vi "Keithley2200series_WaitKeyIccMeas.vi"(0 "VISA Key_In":refnum<visa-resource-name>, 1 "Key":string, 2 "VISA Icc_In":refnum<visa-resource-name>, 3 "error Icc_In":errorcluster) -> (4 "VISA Key_Out":refnum<visa-resource-name>, 6 "Icc, А":string, 7 "Icc, A":dbl, 8 "VISA Icc_Out":refnum<visa-resource-name>, 9 "error Icc_Out":errorcluster)   [LabVIEW 2014]
uses:
  <vilib>/Utility/error.llb/whitespace.ctl
  C:/Users/rad/Desktop/Keithley 2200 Series Power Supplies Ver 1.2 (LV2009)/Keithley 2200 Series/Keithley 2200 Series.lvlib
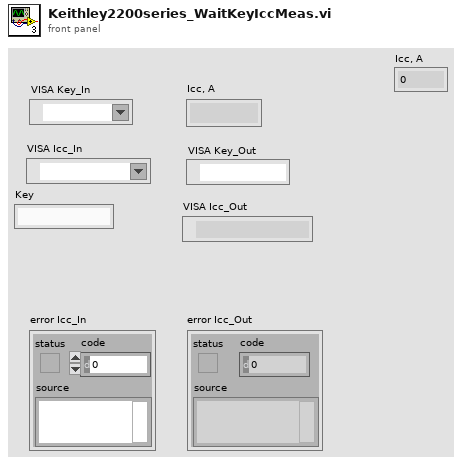
[diagram p1: front panel]
types:
  T1 = typedef "whitespace.ctl" = u16
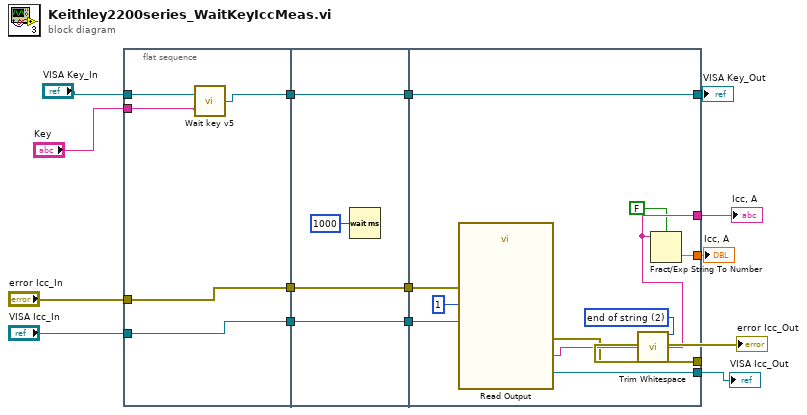
[diagram p0: block diagram]
diagram:
  n1 = flat-sequence {
    tunnel: [w16] -> w6
    tunnel: "VISA Key_In" -> [w18]
    tunnel: [w20] -> w4
    tunnel: "error Icc_In" -> [w20]
    tunnel: [w19] -> w2
    tunnel: "VISA Icc_In" -> [w19]
    tunnel: "Key" -> [w17]
    tunnel: w6 -> [w24]
    tunnel: [w24] -> w5
    tunnel: w4 -> [w23]
    tunnel: [w23] -> w3
    tunnel: w2 -> [w22]
    tunnel: [w22] -> w1
    tunnel: [w32] -> w11
    tunnel: w5 -> [w32]
    tunnel: w3 -> [w31]
    tunnel: w1 -> [w30]
    tunnel: [w29] -> w14
    tunnel: [w28] -> w15
    tunnel: [w27] -> w9
    tunnel: [w26] -> w8
    frame #0 {
      n2 = call "Wait key v5.vi"("Key"=w17, "VISA Refnum in"=w18) -> ("VISA Refnum out"=w16:refnum<visa-resource-name>)
    }
    frame #1 {
      n3 = Wait (ms)(milliseconds to wait=u32 1000) -> ()  [unwired: 1 out]
    }
    frame #2 {
      w34 = T1 2 items=["both", "start of string", "end of string"] ("location (both)")
      n4 = call "Read Output.vi"("VISA resource name"=w30, "Measurement Function (0:Voltage)"=1, "error in (no error)"=w31) -> ("VISA resource name out"=w29:refnum<visa-resource-name>, "Measurement"=w33:string, "error out"=w28:errorcluster)  [unwired: 10 in]
      n5 = call <vilib>:"Trim Whitespace.vi"("string"=w33, "location (both)"=w34) -> ("trimmed string"=w27:string)
      n6 = Fract/Exp String To Number(use system decimal point (T)=FALSE, string=w27) -> (number=w26:dbl)  [unwired: 2 in, 1 out]
    }
  }
  "VISA Key_Out" <- w11
  "VISA Icc_Out" <- w14
  "error Icc_Out" <- w15
  "Icc, А" <- w9
  "Icc, A" <- w8
